vi "IgnoreItemsInPrivateScope.vi"(8 "error in (no error)":errorcluster, 10 "Ignore Items In Private Scope (T)":bool=TRUE, 11 "Whitelist in":refnum<class "Whitelist.lvclass">) -> (0 "error out":errorcluster, 3 "Whitelist out":refnum<class "Whitelist.lvclass">)   [LabVIEW 2017, in "Whitelist.lvclass"]
doc: "If enabled, elements in private scope will be ignored when including libraries."
uses:
  Whitelist.lvclass
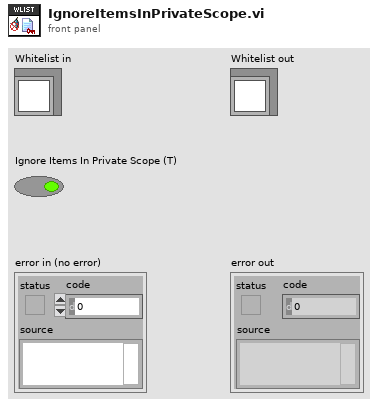
[diagram p1: front panel]
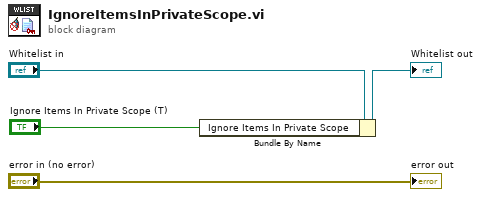
[diagram p0: block diagram]
diagram:
  n1 = Bundle By Name(cluster="Whitelist in", "Ignore Items In Private Scope"="Ignore Items In Private Scope (T)") -> (→"Whitelist out":refnum<class "Whitelist.lvclass">)
  "error out" <- "error in (no error)"
